vi "Calculate Vertex Array.vi"(8 "error in (no error)":errorcluster, 9 "Coordinates System":enum16{"Cartesian", "Cylindrical", "Spherical"}(ring)=enum."Spherical", 10 "3D Quiver Datatype.lvclass in":refnum<class "3D Quiver Datatype.lvclass">, 11 "Plot Representation In":T1) -> (0 "error out":errorcluster, 1 "Dup Coordinates System":enum16{"Cartesian", "Cylindrical", "Spherical"}(ring)=enum."Spherical", 2 "3D Quiver Datatype.lvclass out":refnum<class "3D Quiver Datatype.lvclass">, 3 "Plot Representation Out":T1)   [LabVIEW 2020, in "3D Quiver Datatype.lvclass"]
uses:
  <vilib>/Math Plots/3D Math Plots/3D Quiver/3D Quiver Datatype/3D Quiver Datatype.lvclass
  <vilib>/Math Plots/3D Math Plots/3D Plot/3D Plot/Typedef/Plot Representation.ctl
  <vilib>/Math Plots/3D Math Plots/3D Plot/3D Plot/Typedef/Range Clusters.ctl
  <vilib>/Math Plots/3D Math Plots/3D Plot/3D Plot/Typedef/Mesh Data.ctl
  <vilib>/Math Plots/3D Math Plots/3D Quiver/3D Quiver Datatype/3D Quiver Datatype.lvclass/3D Quiver Datatype.ctl
  <vilib>/Math Plots/3D Math Plots/3D Plot/3D Plot Datatype/3D Plot Datatype.lvclass
  <vilib>/Math Plots/3D Math Plots/3D Plot/3D Plot/3D Plot.lvclass
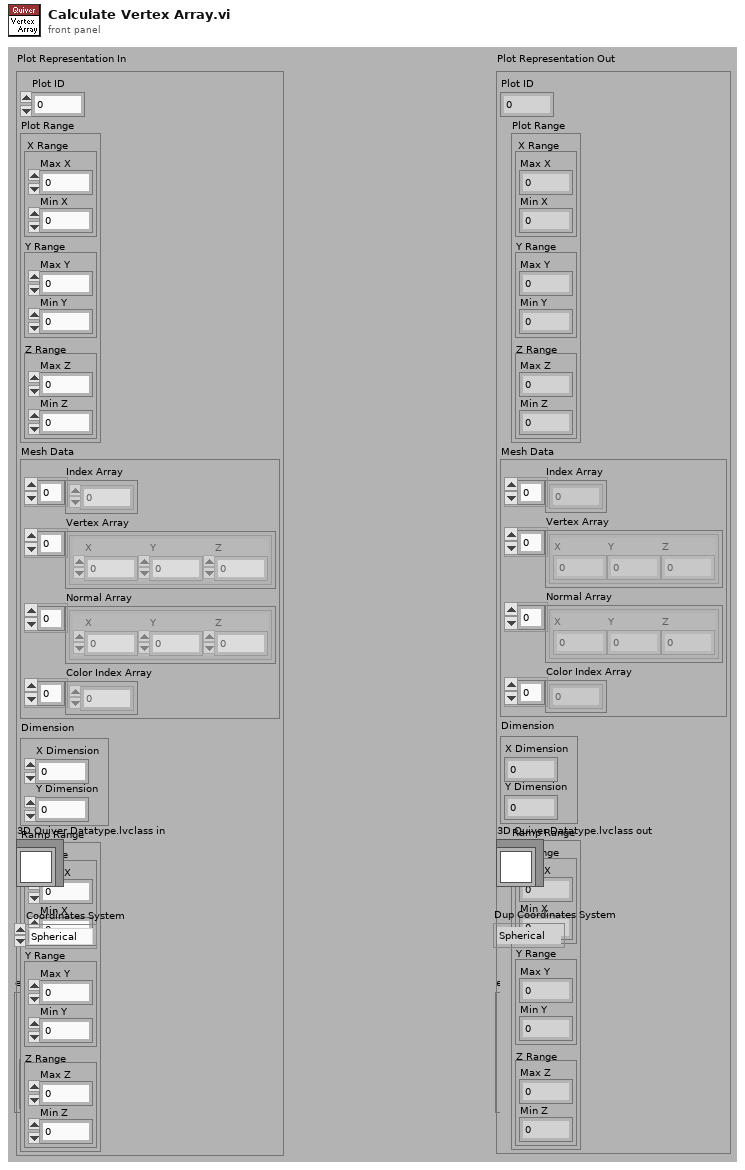
[diagram p1: front panel]
types:
  T1 = typedef "3D Plot.lvclass/Plot Representation.ctl" = cluster{"Plot ID":i32, "Plot Range":T2, "Mesh Data":T3, "Dimension":cluster{"X Dimension":i32, "Y Dimension":i32}, "Ramp Range":T2}
  T2 = typedef "3D Plot.lvclass/Range Clusters.ctl" = cluster{"X Range":cluster{"Max X":sgl, "Min X":sgl}, "Y Range":cluster{"Max Y":sgl, "Min Y":sgl}, "Z Range":cluster{"Max Z":sgl, "Min Z":sgl}}
  T3 = typedef "3D Plot.lvclass/Mesh Data.ctl" = cluster{"Index Array":u32[], "Vertex Array":cluster{"X":sgl, "Y":sgl, "Z":sgl}[], "Normal Array":cluster{"X":sgl, "Y":sgl, "Z":sgl}[], "Color Index Array":i32[]}
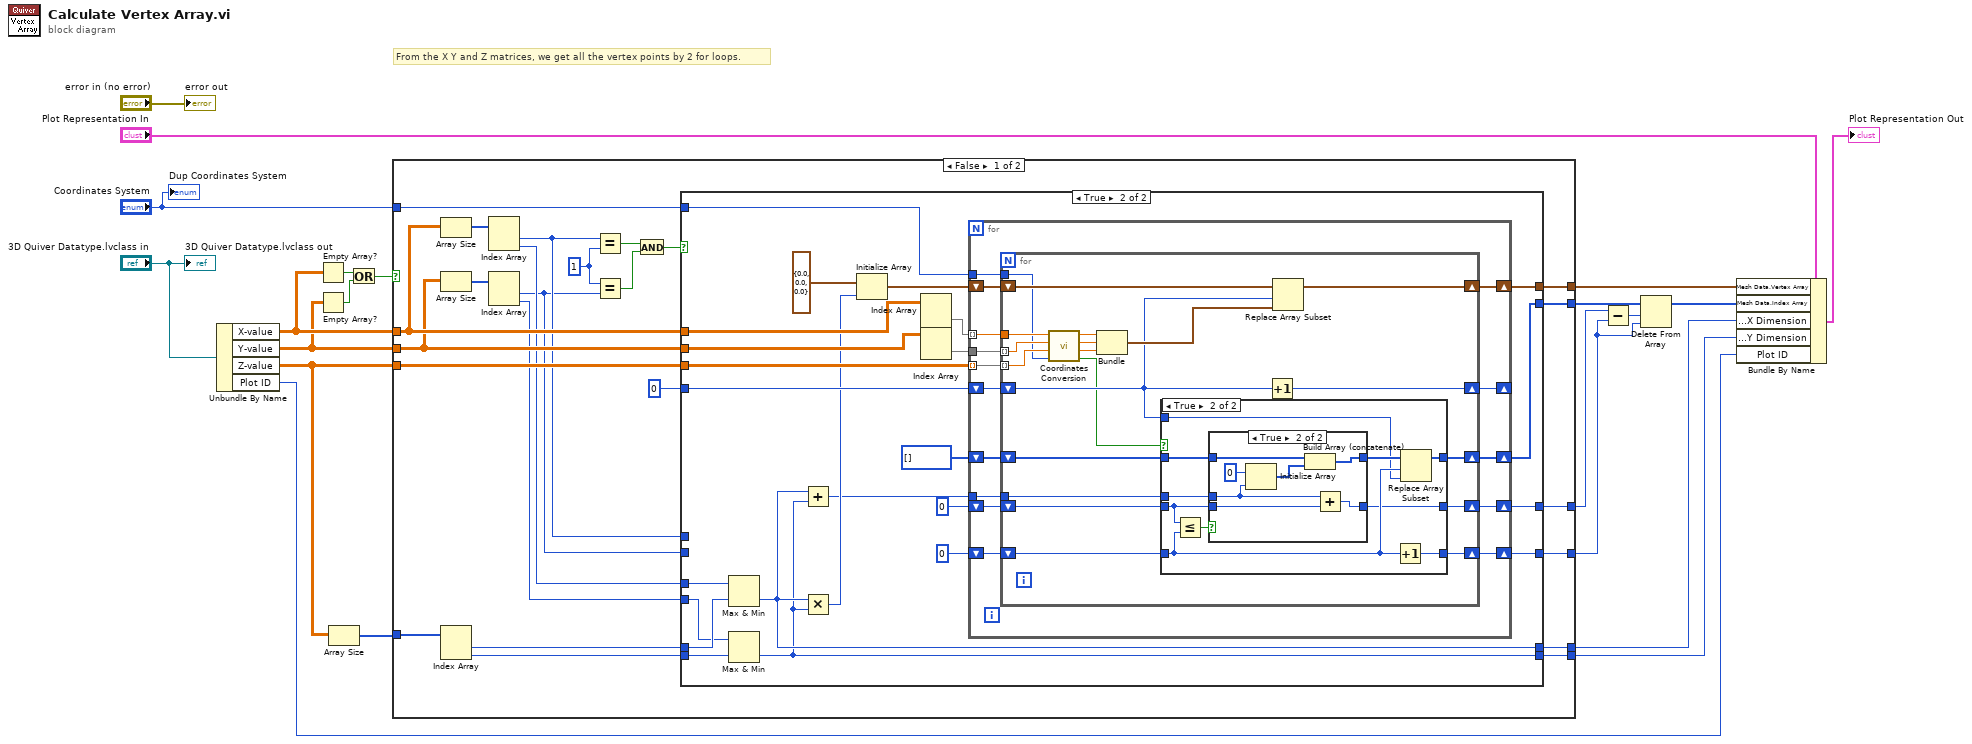
[diagram p0: block diagram]
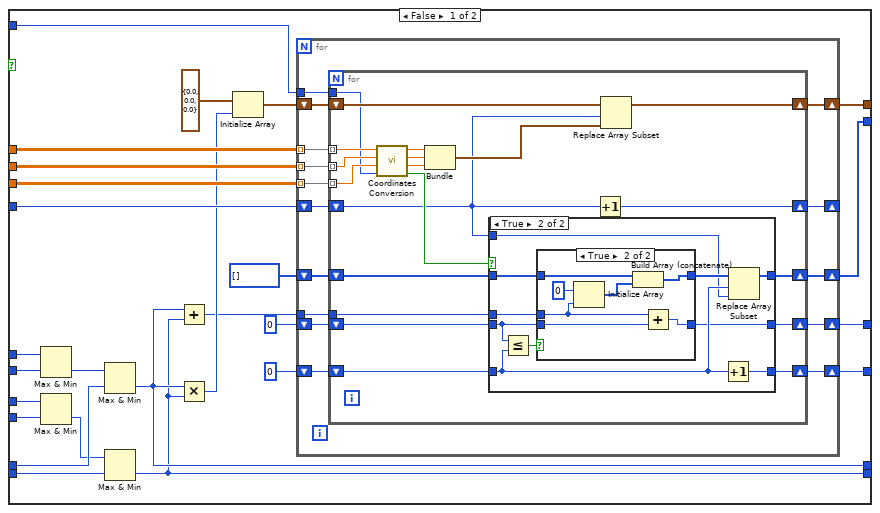
[diagram p2: hidden frame]
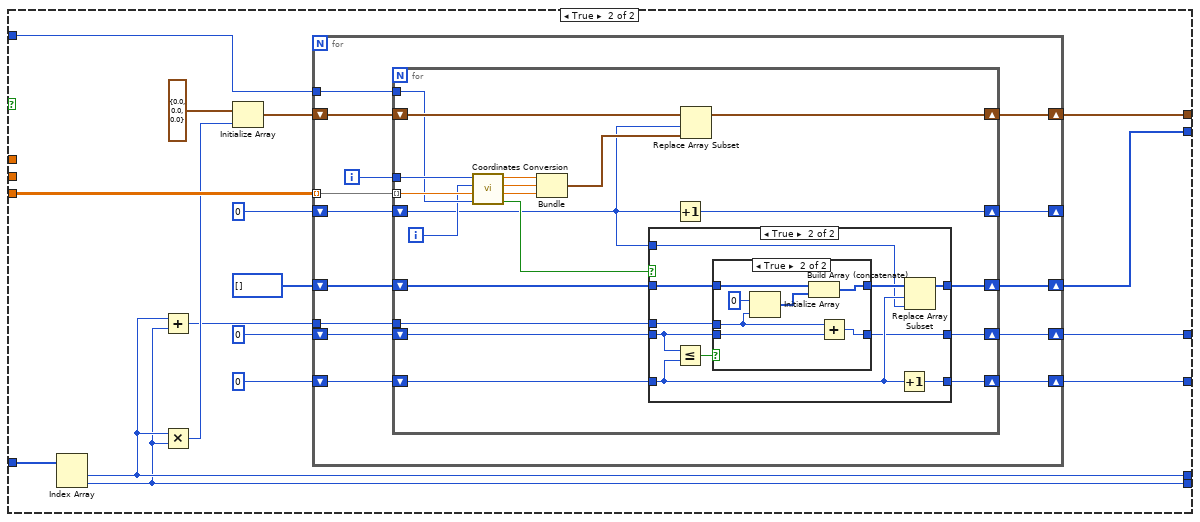
[diagram p7: hidden frame]
diagram:
  # "From the X Y and Z matrices, we get all the vertex points by 2 for loops."
  n1 = Unbundle By Name("3D Quiver Datatype.lvclass in") -> ("X-value"=w3:sgl[][], "Y-value"=w2:sgl[][], "Z-value"=w10:sgl[][], "Plot ID"=w15:i32)
  n2 = Empty Array?(array=w3) -> (empty?=w17:bool)
  n3 = Empty Array?(array=w2) -> (empty?=w16:bool)
  n4 = Array Size(array=w10) -> (size(s)=w9:i32[])
  n5 = Or(x=w17, y=w16) -> (x .or. y?=w1:bool)
  n6 = case shown="False" w1 {
    tunnel: [w33 w226] -> w8
    tunnel: w9 -> [w40 w225]
    tunnel: w10 -> [w35 w224]
    tunnel: "Coordinates System" -> [w38 w223]
    tunnel: [w28 w215] -> w5
    tunnel: [w27 w214] -> w4
    tunnel: w3 -> [w37 _]
    tunnel: w2 -> [w36 _]
    tunnel: [w24 w211] -> w14
    tunnel: [w23 w212] -> w6
    tunnel: [w22 w210] -> w13
    frame False {
      w43 = 1 ("x")
      n7 = Array Size(array=w37) -> (size(s)=w45:i32[])
      n8 = Array Size(array=w36) -> (size(s)=w44:i32[])
      n9 = Index Array(array=w40) -> (element #1=w31:i32, element #2=w29:i32)  [unwired: 2 in]
      n10 = Index Array(array=w45) -> (element #1=w26:i32, element #2=w32:i32)  [unwired: 2 in]
      n11 = Index Array(array=w44) -> (element #1=w25:i32, element #2=w30:i32)  [unwired: 2 in]
      n12 = Equal?(x=w26, y=w43) -> (x = y?=w42:bool)
      n13 = Equal?(x=w43, y=w25) -> (x = y?=w41:bool)
      n14 = And(x=w42, y=w41) -> (x .and. y?=w39:bool)
      n15 = case shown="True" w39 {
        tunnel: w38 -> [w71 w152]
        tunnel: w37 -> [w70 w148]
        tunnel: w36 -> [w69 w147]
        tunnel: w35 -> [w68 w149]
        tunnel: 0 -> [w67 w150]
        tunnel: [w66 w151] -> w33
        tunnel: w32 -> [w61 w142]
        tunnel: w31 -> [w58 w141]
        tunnel: w30 -> [w60 w140]
        tunnel: w29 -> [w56 w139]
        tunnel: [w52 w135] -> w28
        tunnel: [w51 w134] -> w27
        tunnel: w26 -> [w63 _]
        tunnel: w25 -> [w62 _]
        tunnel: [w48 w131] -> w24
        tunnel: [w47 w130] -> w23
        tunnel: [w46 w129] -> w22
        frame False {
          n16 = Max & Min(x=w63, y=w62) -> (min(x,y)=w59:i32)  [unwired: 1 out]
          n17 = Max & Min(x=w61, y=w60) -> (min(x,y)=w57:i32)  [unwired: 1 out]
          n18 = Max & Min(x=w59, y=w58) -> (min(x,y)=w52:i32)  [unwired: 1 out]
          n19 = Max & Min(x=w57, y=w56) -> (min(x,y)=w51:i32)  [unwired: 1 out]
          n20 = Add(x=w52, y=w51) -> (x+y=w50:i32)
          n21 = Multiply(x=w52, y=w51) -> (x*y=w55:i32)
          n22 = Initialize Array(cluster{"X":sgl, "Y":sgl, "Z":sgl} {"X"=0.0, "Y"=0.0, "Z"=0.0} ("3D Point"), w55) -> (w64:cluster{"X":sgl, "Y":sgl, "Z":sgl}[])
          n23 = for {
            shift-right: [w85] -> w66
            shift-left: w64 -> [w86]
            tunnel: w68 -> [w84] mode=indexing
            tunnel: w70 -> [w82] mode=indexing
            tunnel: w69 -> [w83] mode=indexing
            tunnel: w71 -> [w81]
            shift-right: [w79] -> _
            shift-left: w67 -> [w80]
            shift-right: [w77] -> w48
            shift-left: u32[] [] -> [w78]
            shift-right: [w75] -> w46
            shift-left: 0 -> [w73]
            shift-right: [w76] -> w47
            shift-left: 0 -> [w74]
            tunnel: w50 -> [w72]
            n24 = for {
              tunnel: w84 -> [w102] mode=indexing
              shift-right: [w106] -> w85
              shift-left: w86 -> [w105]
              tunnel: w83 -> [w103] mode=indexing
              tunnel: w82 -> [w104] mode=indexing
              tunnel: w81 -> [w98]
              shift-right: [w96] -> w79
              shift-left: w80 -> [w92]
              shift-right: [w95] -> w77
              shift-left: w78 -> [w94]
              shift-right: [w91] -> w76
              shift-left: w74 -> [w88]
              shift-right: [w90] -> w75
              shift-left: w73 -> [w89]
              tunnel: w72 -> [w87]
              n25 = call <vilib>:"Coordinates Conversion.vi"("Coordinates System"=w98, "Z in"=w102, "Y in"=w103, "X in"=w104) -> ("NaN?"=w93:bool, "Z out"=w99:sgl, "Y out"=w100:sgl, "X out"=w101:sgl)  [unwired: 4 out]
              n26 = Bundle("X out"=w101, "Y out"=w100, "Z out"=w99) -> (w97:cluster{"X out":sgl, "Y out":sgl, "Z out":sgl})  [unwired: 1 out]
              n27 = case shown="True" w93 {
                tunnel: w94 -> [w109 w117]
                tunnel: [w109 w113] -> w95
                tunnel: w92 -> [_ w114]
                tunnel: w89 -> [w108 w115]
                tunnel: [w108 w119] -> w90
                tunnel: w88 -> [w107 w111]
                tunnel: [w107 w112] -> w91
                tunnel: w87 -> [_ w110]
                frame False {
                }
                frame True {
                  n28 = Less Or Equal?(x=w111, y=w115) -> (x <= y?=w118:bool)
                  n29 = case shown="True" w118 {
                    tunnel: w117 -> [w121 w128]
                    tunnel: [w121 w127] -> w116
                    tunnel: [w120 w123] -> w112
                    tunnel: w111 -> [w120 w124]
                    tunnel: w110 -> [_ w122]
                    frame False {
                    }
                    frame True {
                      n30 = Initialize Array(u32 0, w122) -> (w125:u32[])
                      n31 = Build Array (concatenate)(w128, w125) -> (w127:u32[])
                      n32 = Add(x=w122, y=w124) -> (x+y=w123:i32)
                    }
                  }
                  n33 = Increment(x=w115) -> (x+1=w119:i32)
                  n34 = Replace Array Subset(array=w116, new element=w114, index=w115) -> (w113:u32[])
                }
              }
              n35 = Increment(x=w92) -> (x+1=w96:i32)
              n36 = Replace Array Subset(array=w105, new element=w97, index=w92) -> (w106:cluster{"X":sgl, "Y":sgl, "Z":sgl}[])
            }
          }
        }
        frame True {
          n37 = Max & Min(x=w142, y=w141) -> (min(x,y)=w135:i32)  [unwired: 1 out]
          n38 = Max & Min(x=w140, y=w139) -> (min(x,y)=w134:i32)  [unwired: 1 out]
          n39 = Add(x=w135, y=w134) -> (x+y=w133:i32)
          n40 = Multiply(x=w135, y=w134) -> (x*y=w138:i32)
          n41 = Initialize Array(cluster{"X":sgl, "Y":sgl, "Z":sgl} {"X"=0.0, "Y"=0.0, "Z"=0.0} ("3D Point"), w138) -> (w143:cluster{"X":sgl, "Y":sgl, "Z":sgl}[])
          n42 = Index Array(array=w148) -> (element=w145:sgl[])  [unwired: 2 in]
          n43 = Index Array(array=w147) -> (element=w146:sgl[])  [unwired: 2 in]
          n44 = for {
            shift-right: [w166] -> w151
            shift-left: w143 -> [w167]
            tunnel: w149 -> [w165] mode=indexing
            tunnel: w145 -> [w163] mode=indexing
            tunnel: w146 -> [w164]
            tunnel: w152 -> [w162]
            shift-right: [w160] -> _
            shift-left: w150 -> [w161]
            shift-right: [w158] -> w131
            shift-left: u32[] [] -> [w159]
            shift-right: [w155] -> w129
            shift-left: 0 -> [w156]
            shift-right: [w154] -> w130
            shift-left: 0 -> [w157]
            tunnel: w133 -> [w153]
            n45 = for {
              tunnel: w165 -> [w183] mode=indexing
              shift-right: [w187] -> w166
              shift-left: w167 -> [w186]
              tunnel: w164 -> [w184] mode=indexing
              tunnel: w163 -> [w185]
              tunnel: w162 -> [w179]
              shift-right: [w177] -> w160
              shift-left: w161 -> [w174]
              shift-right: [w175] -> w158
              shift-left: w159 -> [w176]
              shift-right: [w171] -> w155
              shift-left: w156 -> [w172]
              shift-right: [w169] -> w154
              shift-left: w157 -> [w170]
              tunnel: w153 -> [w168]
              n46 = call <vilib>:"Coordinates Conversion.vi"("Coordinates System"=w179, "Z in"=w183, "Y in"=w184, "X in"=w185) -> ("NaN?"=w173:bool, "Z out"=w180:sgl, "Y out"=w181:sgl, "X out"=w182:sgl)  [unwired: 4 out]
              n47 = Bundle("X out"=w182, "Y out"=w181, "Z out"=w180) -> (w178:cluster{"X out":sgl, "Y out":sgl, "Z out":sgl})  [unwired: 1 out]
              n48 = case shown="True" w173 {
                tunnel: w176 -> [w190 w198]
                tunnel: [w190 w194] -> w175
                tunnel: w174 -> [_ w195]
                tunnel: w172 -> [w189 w196]
                tunnel: [w189 w200] -> w171
                tunnel: w170 -> [w188 w192]
                tunnel: [w188 w193] -> w169
                tunnel: w168 -> [_ w191]
                frame False {
                }
                frame True {
                  n49 = Less Or Equal?(x=w192, y=w196) -> (x <= y?=w199:bool)
                  n50 = case shown="True" w199 {
                    tunnel: w198 -> [w202 w209]
                    tunnel: [w202 w208] -> w197
                    tunnel: [w201 w204] -> w193
                    tunnel: w192 -> [w201 w205]
                    tunnel: w191 -> [_ w203]
                    frame False {
                    }
                    frame True {
                      n51 = Initialize Array(u32 0, w203) -> (w206:u32[])
                      n52 = Build Array (concatenate)(w209, w206) -> (w208:u32[])
                      n53 = Add(x=w203, y=w205) -> (x+y=w204:i32)
                    }
                  }
                  n54 = Increment(x=w196) -> (x+1=w200:i32)
                  n55 = Replace Array Subset(array=w197, new element=w195, index=w196) -> (w194:u32[])
                }
              }
              n56 = Increment(x=w174) -> (x+1=w177:i32)
              n57 = Replace Array Subset(array=w186, new element=w178, index=w174) -> (w187:cluster{"X":sgl, "Y":sgl, "Z":sgl}[])
            }
          }
        }
      }
    }
    frame True {
      n58 = Index Array(array=w225) -> (element #1=w215:i32, element #2=w214:i32)  [unwired: 2 in]
      n59 = Add(x=w215, y=w214) -> (x+y=w213:i32)
      n60 = Multiply(x=w215, y=w214) -> (x*y=w220:i32)
      n61 = Initialize Array(cluster{"X":sgl, "Y":sgl, "Z":sgl} {"X"=0.0, "Y"=0.0, "Z"=0.0} ("3D Point"), w220) -> (w221:cluster{"X":sgl, "Y":sgl, "Z":sgl}[])
      n62 = for {
        shift-right: [w239] -> w226
        shift-left: w221 -> [w240]
        tunnel: w224 -> [w238] mode=indexing
        tunnel: w223 -> [w237]
        shift-right: [w235] -> _
        shift-left: 0 -> [w236]
        shift-right: [w232] -> w211
        shift-left: u32[] [] -> [w233]
        shift-right: [w229] -> w212
        shift-left: 0 -> [w231]
        shift-right: [w228] -> w210
        shift-left: 0 -> [w230]
        tunnel: w213 -> [w227]
        i -> [w234]
        n63 = for {
          tunnel: w238 -> [w257] mode=indexing
          shift-right: [w260] -> w239
          shift-left: w240 -> [w259]
          tunnel: w234 -> [w258]
          tunnel: w237 -> [w253]
          shift-right: [w251] -> w235
          shift-left: w236 -> [w247]
          shift-right: [w249] -> w232
          shift-left: w233 -> [w242]
          shift-right: [w243] -> w228
          shift-left: w230 -> [w245]
          shift-right: [w244] -> w229
          shift-left: w231 -> [w246]
          tunnel: w227 -> [w241]
          i -> [w250]
          n64 = call <vilib>:"Coordinates Conversion.vi"("Coordinates System"=w253, "Z in"=w257, "Y in"=w250, "X in"=w258) -> ("NaN?"=w248:bool, "Z out"=w254:sgl, "Y out"=w255:sgl, "X out"=w256:sgl)  [unwired: 4 out]
          n65 = Bundle("X out"=w256, "Y out"=w255, "Z out"=w254) -> (w252:cluster{"X out":sgl, "Y out":sgl, "Z out":sgl})  [unwired: 1 out]
          n66 = case shown="True" w248 {
            tunnel: w242 -> [w263 w271]
            tunnel: [w263 w267] -> w249
            tunnel: w247 -> [_ w268]
            tunnel: w245 -> [w262 w269]
            tunnel: [w262 w273] -> w243
            tunnel: w246 -> [w261 w265]
            tunnel: [w261 w266] -> w244
            tunnel: w241 -> [_ w264]
            frame False {
            }
            frame True {
              n67 = Less Or Equal?(x=w265, y=w269) -> (x <= y?=w272:bool)
              n68 = case shown="True" w272 {
                tunnel: w271 -> [w275 w282]
                tunnel: [w275 w281] -> w270
                tunnel: [w274 w277] -> w266
                tunnel: w265 -> [w274 w278]
                tunnel: w264 -> [_ w276]
                frame False {
                }
                frame True {
                  n69 = Initialize Array(u32 0, w276) -> (w279:u32[])
                  n70 = Build Array (concatenate)(w282, w279) -> (w281:u32[])
                  n71 = Add(x=w276, y=w278) -> (x+y=w277:i32)
                }
              }
              n72 = Increment(x=w269) -> (x+1=w273:i32)
              n73 = Replace Array Subset(array=w270, new element=w268, index=w269) -> (w267:u32[])
            }
          }
          n74 = Increment(x=w247) -> (x+1=w251:i32)
          n75 = Replace Array Subset(array=w259, new element=w252, index=w247) -> (w260:cluster{"X":sgl, "Y":sgl, "Z":sgl}[])
        }
      }
    }
  }
  n76 = Subtract(x=w6, y=w13) -> (x-y=w12:i32)
  n77 = Delete From Array(array=w14, length=w12, index=w13) -> (array with subset deleted=w7:u32[])  [unwired: 1 out]
  n78 = Bundle By Name(cluster="Plot Representation In", "Mesh Data.Vertex Array"=w8, "Mesh Data.Index Array"=w7, "Dimension.X Dimension"=w5, "Dimension.Y Dimension"=w4, "Plot ID"=w15) -> (→"Plot Representation Out":T1)
  "error out" <- "error in (no error)"
  "3D Quiver Datatype.lvclass out" <- "3D Quiver Datatype.lvclass in"
  "Dup Coordinates System" <- "Coordinates System"
